vi "Op-Download Trace.vi"(8 "error in (no error)":errorcluster, 10 "trace (variable) name":string, 11 "VISA session":refnum<visa-resource-name>) -> (0 "error out":errorcluster, 1 "trace":dbl[](array[numeric]) format="%^.3e", 3 "VISA resource name out":refnum<visa-resource-name>)   [LabVIEW 2016, in "Agilent 415X Series.lvlib"]
doc: "This VI reads trace data from the instrument.\n\nLimited error checking is performed before querying the instrument for data if the ActiveErrorChecking global variable is set to TRUE (see HP 415xA Initialize.vi). This VI varifies the existence of the variable by searching for its name in the variable list.\n\nHP415xA Op. Start-Stop.vi must be run first to acquire a trace."
uses:
  Agilent 415X Series.lvlib
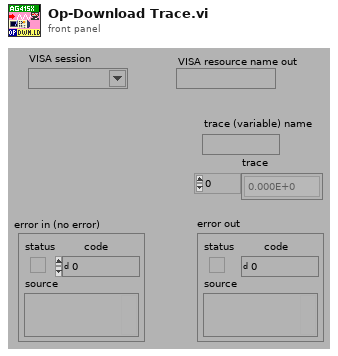
[diagram p1: front panel]
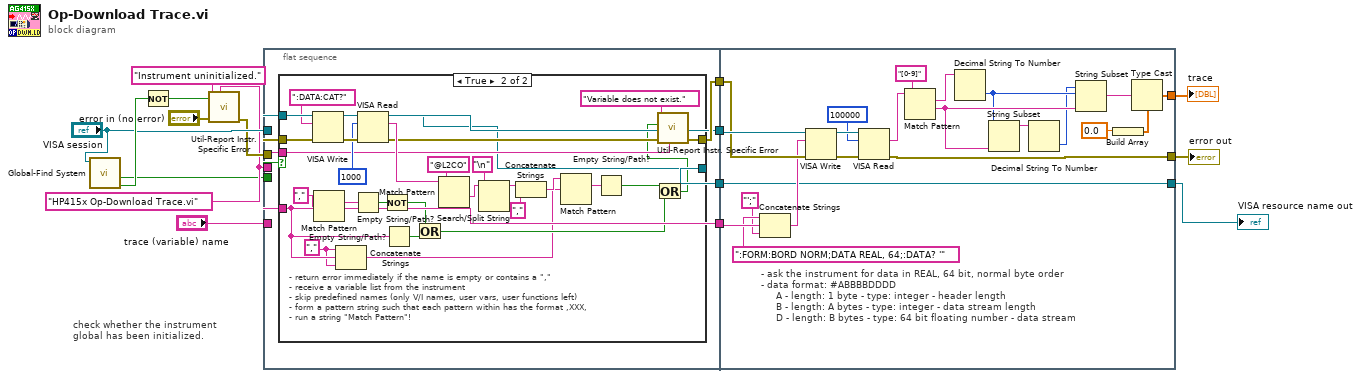
[diagram p0: block diagram]
diagram:
  w10 = "HP415x Op-Download Trace.vi"
  # "check whether the instrument\nglobal has been initialized."
  n1 = call "Global-Find System.vi"("VISA session"="VISA session") -> ("found"=w15:bool, "active error checking"=w9:bool)  [unwired: 3 in, 6 out]
  n2 = Not(x=w15) -> (.not. x?=w14:bool)
  n3 = call "Util-Report Instr. Specific Error.vi"("source"=w10, "error in (no error)"="error in (no error)", "error message"="Instrument uninitialized.", "new error"=w14) -> ("error out"=w11:errorcluster)  [unwired: 6 in, 1 out]
  n4 = flat-sequence {
    tunnel: "VISA session" -> [w18]
    tunnel: [w18] -> w4
    tunnel: w11 -> [w23]
    tunnel: w10 -> [w22]
    tunnel: w9 -> [w21]
    tunnel: "trace (variable) name" -> [w17]
    tunnel: [w17] -> w3
    tunnel: [w19] -> w2
    tunnel: [w20] -> w1
    tunnel: w4 -> [w74]
    tunnel: w3 -> [w72]
    tunnel: [w69] -> w7
    tunnel: [w59] -> w6
    tunnel: [w56] -> w5
    tunnel: w2 -> [w56]
    tunnel: w1 -> [w73]
    frame #0 {
      n5 = case shown="True" w21 {
        tunnel: w18 -> [w24 w55]
        tunnel: w23 -> [w25 w54]
        tunnel: w17 -> [_ w44]
        tunnel: w22 -> [_ w31]
        tunnel: [w25 w32] -> w20
        tunnel: [w24 w26] -> w19
        frame False {
          # "Active Error Checking is OFF"
        }
        frame True {
          w41 = ","
          # "- return error immediately if the name is empty or contains a \",\"\n- receive a variable list from the instrument\n- skip predefined names (only V/I names, user vars, user functions left)\n- form a pattern string such that each pattern within has the format ,XXX,\n- run a string \"Match Pattern\"!"
          n6 = VISA Write(VISA resource name=w55, write buffer=":DATA:CAT?", error in (no error)=w54) -> (VISA resource name out=w49:refnum<visa-resource-name>, error out=w48:errorcluster)  [unwired: 1 out]
          n7 = Match Pattern(string=w44, regular expression=",") -> (match substring=w51:string)  [unwired: 1 in, 3 out]
          n8 = Concatenate Strings(w41, w44, w41) -> (w27:string)
          n9 = Empty String/Path?(string/path=w51) -> (empty?=w50:bool)
          n10 = VISA Read(VISA resource name=w49, byte count=1000, error in (no error)=w48) -> (VISA resource name out=w26:refnum<visa-resource-name>, read buffer=w46:string, error out=w33:errorcluster)  [unwired: 1 out]
          n11 = Not(x=w50) -> (.not. x?=w43:bool)
          n12 = Empty String/Path?(string/path=w44) -> (empty?=w42:bool)
          n13 = Or(x=w43, y=w42) -> (x .or. y?=w35:bool)
          n14 = Match Pattern(string=w46, regular expression="@L2CO") -> (after substring=w40:string)  [unwired: 1 in, 3 out]
          n15 = Search/Split String(string=w40, search string/char (-)="\n") -> (substring before match=w38:string)  [unwired: 1 in, 2 out]
          n16 = Concatenate Strings(w38, ",") -> (w36:string)
          n17 = Match Pattern(string=w36, regular expression=w27) -> (match substring=w34:string)  [unwired: 1 in, 3 out]
          n18 = Empty String/Path?(string/path=w34) -> (empty?=w28:bool)
          n19 = Or(x=w35, y=w28) -> (x .or. y?=w29:bool)
          n20 = call "Util-Report Instr. Specific Error.vi"("source"=w31, "error in (no error)"=w33, "error message"="Variable does not exist.", "new error"=w29) -> ("error out"=w32:errorcluster)  [unwired: 6 in, 1 out]
        }
      }
    }
    frame #1 {
      # "- ask the instrument for data in REAL, 64 bit, normal byte order\n- data format: #ABBBBDDDD \n     A - length: 1 byte - type: integer - header length\n     B - length: A bytes - type: integer - data stream length\n     D - length: B bytes - type: 64 bit floating number - data stream"
      n21 = Concatenate Strings(":FORM:BORD NORM;DATA REAL, 64;:DATA? '", w72, "';") -> (w70:string)
      n22 = VISA Write(VISA resource name=w74, write buffer=w70, error in (no error)=w73) -> (VISA resource name out=w77:refnum<visa-resource-name>, error out=w76:errorcluster)  [unwired: 1 out]
      n23 = VISA Read(VISA resource name=w77, byte count=100000, error in (no error)=w76) -> (read buffer=w57:string, error out=w69:errorcluster)  [unwired: 2 out]
      n24 = Match Pattern(string=w57, regular expression="[0-9]") -> (match substring=w67:string, after substring=w65:string)  [unwired: 1 in, 2 out]
      n25 = Decimal String To Number(string=w67) -> (number=w64:i32)  [unwired: 2 in, 1 out]
      n26 = String Subset(string=w65, length (rest)=w64) -> (substring=w63:string)  [unwired: 1 in]
      n27 = Decimal String To Number(string=w63) -> (number=w62:i32)  [unwired: 2 in, 1 out]
      n28 = String Subset(string=w65, offset (0)=w64, length (rest)=w62) -> (substring=w60:string)
      n29 = Build Array(0.0) -> (w61:dbl[])
      n30 = Type Cast(type=w61, x=w60) -> (*(type *) &x=w59:dbl[])
    }
  }
  "error out" <- w7
  "trace" <- w6
  "VISA resource name out" <- w5
